vi "UDP - Sender - 2 D array.vi"() -> ()   [LabVIEW 2016]
doc: "The UDP protocol differs from TCP in that there is no error-checking with the packets of information that are sent, and thus no guarantee whatsoever that an intended recipient will actually receive a given piece of data.\n\nUDP does offer the ability to \"broadcast\" data across a network--simply specify an IP Address of all ones (255.255.255.255) to attempt to broadcast information network-wide. Keep in mind that routers and other network hardware will generally refuse to forward the broadcast beyond certain points, so the extent of the broadcast will in practice be limited."
panel:
  out "Byte array size":i32
  out "Timeout Error":bool
  in  "Stop":bool
  # "Overview: Demonstrates the use of the UDP functions to send data over a UDP connection.\nInstructions:\n1. Run the VI.\n2. Open Simple UDP - Receiver.vi and follow the instructions on its front panel.\n3. Click Stop to stop the VI."
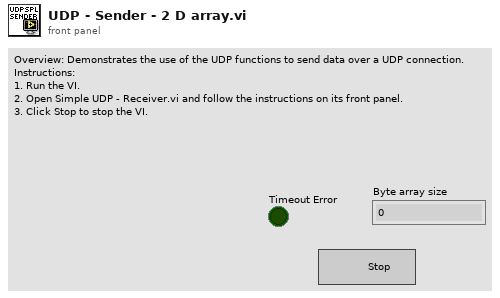
[diagram p1: front panel]
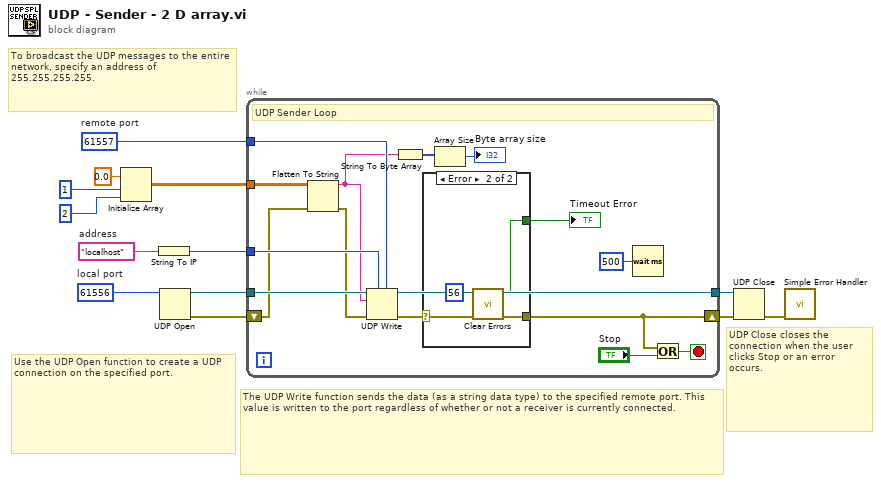
[diagram p0: block diagram]
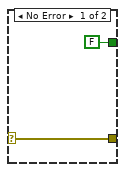
[diagram p2: hidden frame]
diagram:
  w5 = u16 61557  # remote port
  w6 = u16 61556  # local port
  w11 = "localhost"  # address
  # "To broadcast the UDP messages to the entire network, specify an address of 255.255.255.255."
  # "UDP Close closes the connection when the user clicks Stop or an error occurs."
  # "The UDP Write function sends the data (as a string data type) to the specified remote port. This value is written to the port regardless of whether or not a receiver is currently connected."
  # "Use the UDP Open function to create a UDP connection on the specified port."
  n1 = Initialize Array(0.0 ("element"), 1 ("dimension size"), 2 ("dimension size")) -> (w1:dbl[][])
  n2 = String To IP(1:w11) -> (0:w9:u32)
  n3 = UDP Open(11:w6) -> (port=w8:refnum<k16>, 0:w7:errorcluster)  [unwired: 4 in, 1 out]
  n4 = while {
    tunnel: w8 -> [w29]
    tunnel: [w25] -> w13
    tunnel: w9 -> [w24]
    tunnel: w5 -> [w23]
    tunnel: w1 -> [w20]
    shift-right: [w18] -> w12
    shift-left: w7 -> [w22]
    stop <- w28 stop-if-true
    # "UDP Sender Loop"
    n5 = Flatten To String(anything=w20, error in (no error)=w22) -> (data string=w16:string, error out=w21:errorcluster)  [unwired: 2 in, 1 out]
    n6 = UDP Write(address=w24, port or service name=w23, connection ID=w29, data in=w16, 8:w21) -> (error out=w19:errorcluster, 3:w25:refnum<k16>)  [unwired: 1 in]
    n7 = String To Byte Array(string=w16) -> (unsigned byte array=w15:u8[])
    n8 = case shown="Error" w19 {
      selector: w19 -> [w31 w35]
      tunnel: [w31 w33] -> w18
      tunnel: [FALSE ("specific error cleared?") w32] -> w17
      frame No Error {
      }
      frame Error {
        n9 = call <vilib>:"Clear Errors.vi"("error in (no error)"=w35, "specific error code to clear (0: all)"=56) -> ("error out"=w33:errorcluster, "specific error cleared?"=w32:bool)  [unwired: 4 in]
      }
    }
    "Timeout Error" <- w17
    n10 = Array Size(array=w15) -> (size(s)=→"Byte array size":i32)
    n11 = Wait (ms)(milliseconds to wait=u32 500) -> ()  [unwired: 1 out]
    n12 = Or(x=w18, y="Stop") -> (x .or. y?=w28:bool)
  }
  n13 = UDP Close(connection ID=w13, 8:w12) -> (error out=w10:errorcluster)  [unwired: 1 out]
  n14 = call <vilib>:"Simple Error Handler.vi"("error in (no error)"=w10) -> ()  [unwired: 4 in, 5 out]
